vi "Live webcam face tracking.vi"() -> ()   [LabVIEW 2018]
panel:
  out "Image Out 2":T1(plugin-control)
  out "error out":errorcluster
  in  "error in":errorcluster
  out "return value":i32[][](array[numeric])=[[278, 97, 240, 240], [47, 217, 163, 163]]
  in  "File Path":path=path "D:/image.jpg"
  in  "Stop (F)":bool
  out "Image Out":T1(plugin-control)
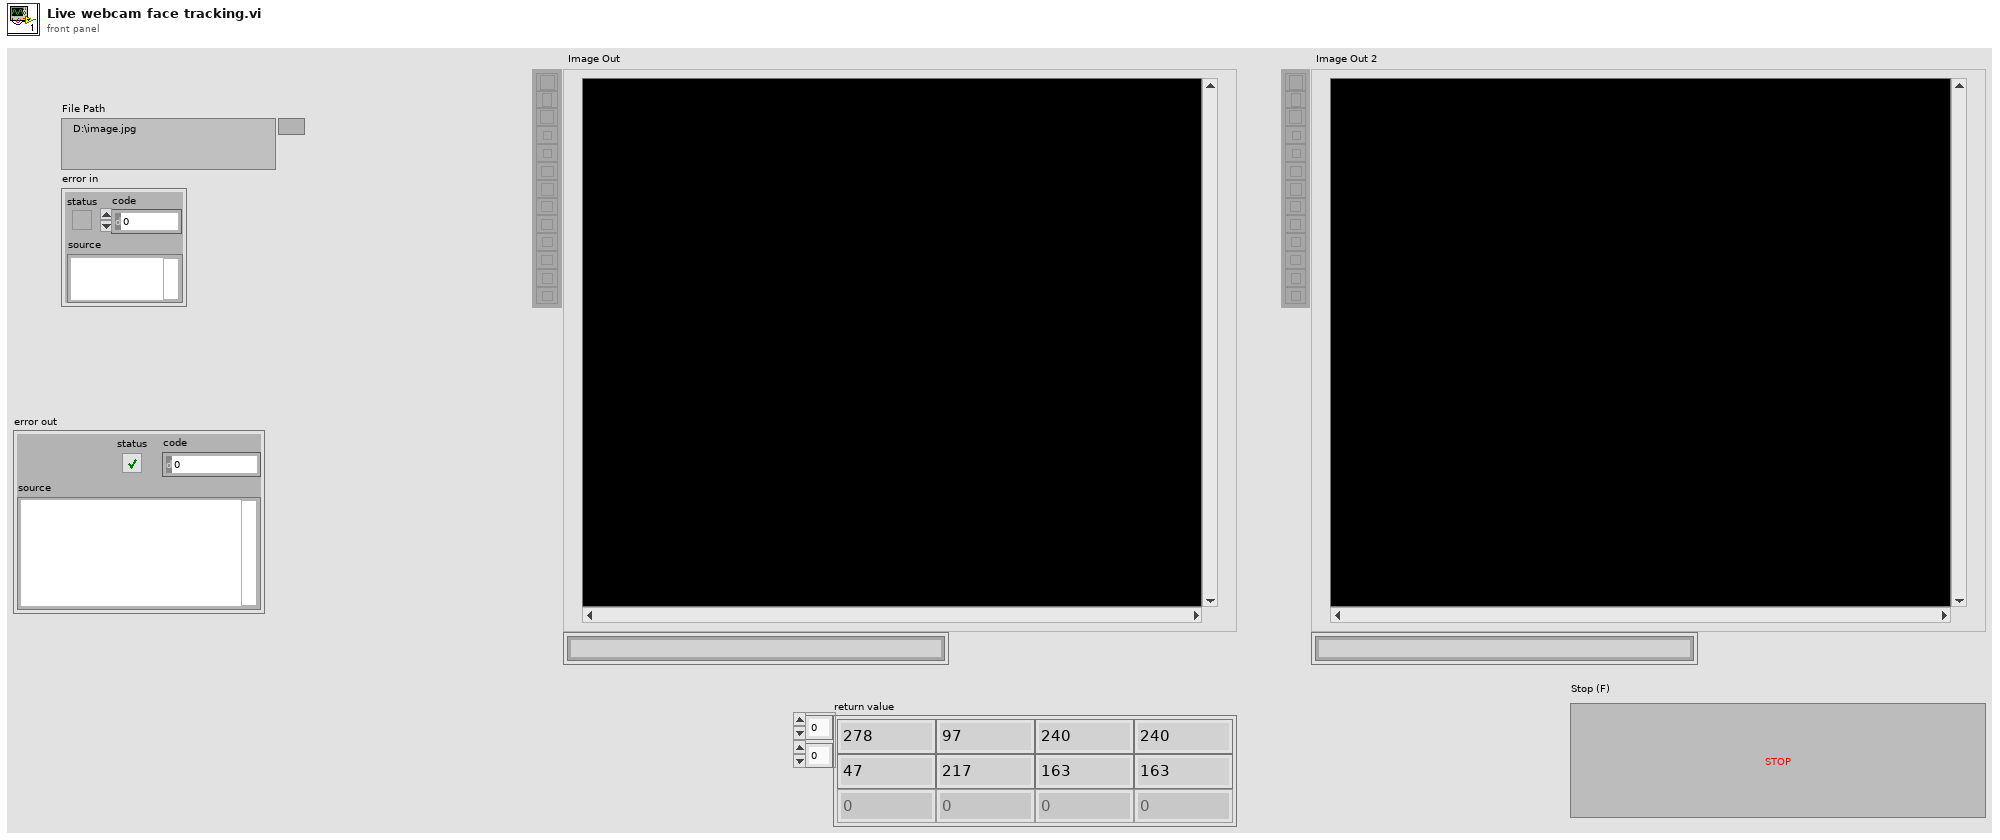
[diagram p1: front panel]
types:
  T1 = typedef "IMAQ Image.ctl" = refnum<image>
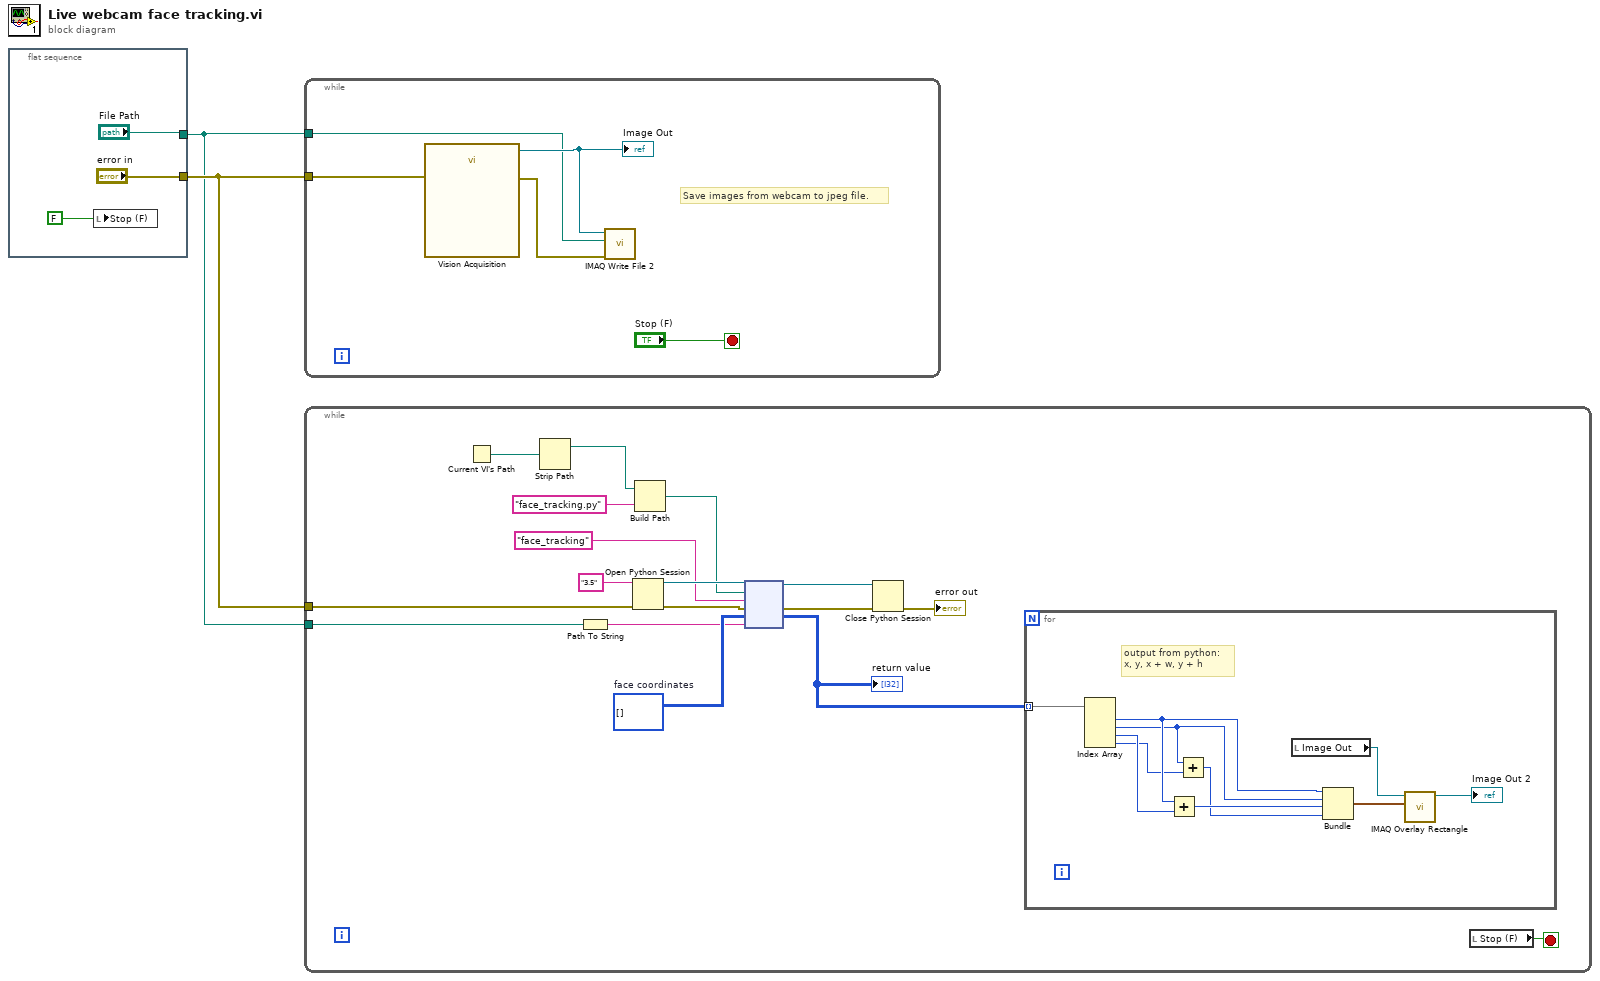
[diagram p0: block diagram]
diagram:
  n1 = flat-sequence {
    tunnel: ["error in"] -> w2
    tunnel: ["File Path"] -> w1
    frame #0 {
      n2 = local write "Stop (F)"(FALSE ("Stop (F)")) -> ()
    }
  }
  n3 = while {
    tunnel: w2 -> [w7]
    tunnel: w1 -> [w6]
    stop <- "Stop (F)" stop-if-true
    # "Save images from webcam to jpeg file."
    n4 = call "Vision Acquisition"("error in"=w7) -> ("Image Out"=w10:T1, "error out"=w9:errorcluster)  [unwired: 24 in, 1 out]
    "Image Out" <- w10
    n5 = call-poly "IMAQ Write File 2"("error in (no error)"=w9, "File Path"=w6, "Image"=w10) -> ()  [unwired: 7 in, 2 out]
  }
  n6 = while {
    tunnel: w2 -> [w21]
    tunnel: w1 -> [w11]
    stop <- w20 stop-if-true
    w22 = i32[][] []  # face coordinates
    n7 = Current VI's Path() -> (path=w16:path)
    n8 = Strip Path(path=w16) -> (stripped path=w14:path)  [unwired: 1 out]
    n9 = Path To String(path=w11) -> (string=w12:string)
    n10 = Open Python Session(python version="3.5" ("Python version"), 3:w21) -> (session out=w26:refnum<k35>, error out=w25:errorcluster)  [unwired: 1 in]
    n11 = Build Path(base path=w14, name or relative path="face_tracking.py") -> (appended path=w13:path)
    n12 = node(w26, w13, "face_tracking" ("function name"), w25, w22, w12) -> (w24:refnum<k35>, w23:errorcluster, w17:i32[][])  [unwired: 1 in, 2 out]
    "return value" <- w17
    n13 = Close Python Session(session in=w24, error in=w23) -> (11:→"error out":errorcluster)
    n14 = for {
      tunnel: w17 -> [w37] mode=indexing
      # "output from python:\nx, y, x + w, y + h"
      n15 = Index Array(array=w37) -> (element #1=w34:i32, element #2=w29:i32, element #3=w33:i32, element #4=w31:i32)  [unwired: 4 in]
      n16 = Add(x=w34, y=w33) -> (x+y=w32:i32)
      n17 = Add(x=w29, y=w31) -> (x+y=w30:i32)
      n18 = local read "Image Out"() -> (w36:T1)
      n19 = Bundle(w34, w29, w32, w30) -> (w28:cluster{i32, i32, i32, i32})  [unwired: 1 in]
      n20 = call "IMAQ Overlay Rectangle"("Rectangle"=w28, "Image"=w36) -> ("Image Out"=→"Image Out 2":T1)  [unwired: 8 in, 1 out]
    }
    n21 = local read "Stop (F)"() -> (w20:bool)
  }
